vi "Script 3.vi"() -> ()   [LabVIEW 2020]
uses:
  <vilib>/Utility/miscctls.llb/LVRectTypeDef.ctl
  <vilib>/Utility/miscctls.llb/LVPositionTypeDef.ctl
  _csmHelper/CSM-Helper.lvclass/CSM-Helper.ctl
  _csmHelper/Properties/Read Case Structure Ref.vi
  _csmHelper/API/Create From VI Reference.vi
  _csmHelper/API/Start Undo.vi
  _csmHelper/Properties/Read Block Diagram Ref.vi
  _csmHelper/API/Destroy.vi
  _csmHelper/API/Connect StateQ Wire If not Connected.vi
  _csmHelper/API/Connect Internal Data Wire If not Connected.vi
  _csmHelper/API/Set Error Tunnel Use Default If not Connected.vi
  _csmHelper/API/Get CaseFrame Reference By CaseName.vi
  _csmHelper/API/Stop Undo.vi
  _csmHelper/CSM-Helper.lvclass
panel:
  in  "Top":i16
  in  "Left":i16
  out "Bounds:Area Height 2":u32
  out "Bounds:Area Width 2":u32
  out "Bounds:Area Width":u32
  out "Bounds:Area Height":u32
  in  "element":string="UI: Cursor Set"
  out "index of element":i32[](array[numeric])
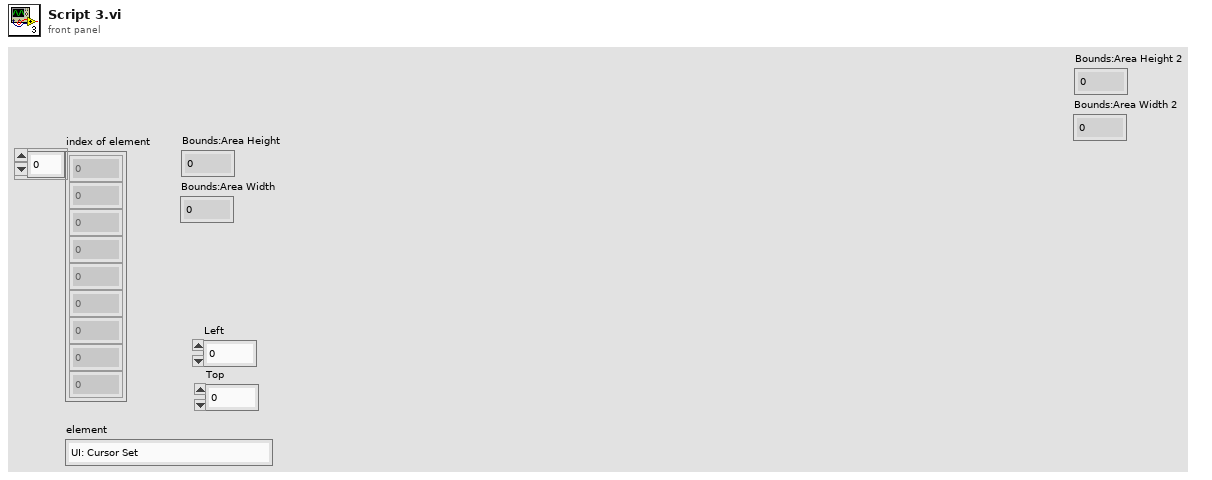
[diagram p1: front panel]
types:
  T1 = typedef "LVPositionTypeDef.ctl" = cluster{"Left":i32, "Top":i32}
  T2 = typedef "LVRectTypeDef.ctl" = cluster{"Left":i16, "Top":i16, "Right":i16, "Bottom":i16}
  T3 = cluster{"InternalData":refnum<vi>, "CSM Name":refnum<vi>, "Last Resp":refnum<vi>, "Remaining State":refnum<vi>, "Arguments":refnum<vi>, "Response Source":refnum<vi>, "Source CSM":refnum<vi>, "Selector":refnum<vi>, "Error":refnum<vi>}
  T4 = cluster{"InternalData":refnum<vi>, "Resp":refnum<vi>, "Remaining State":refnum<vi>, "Error":refnum<vi>}
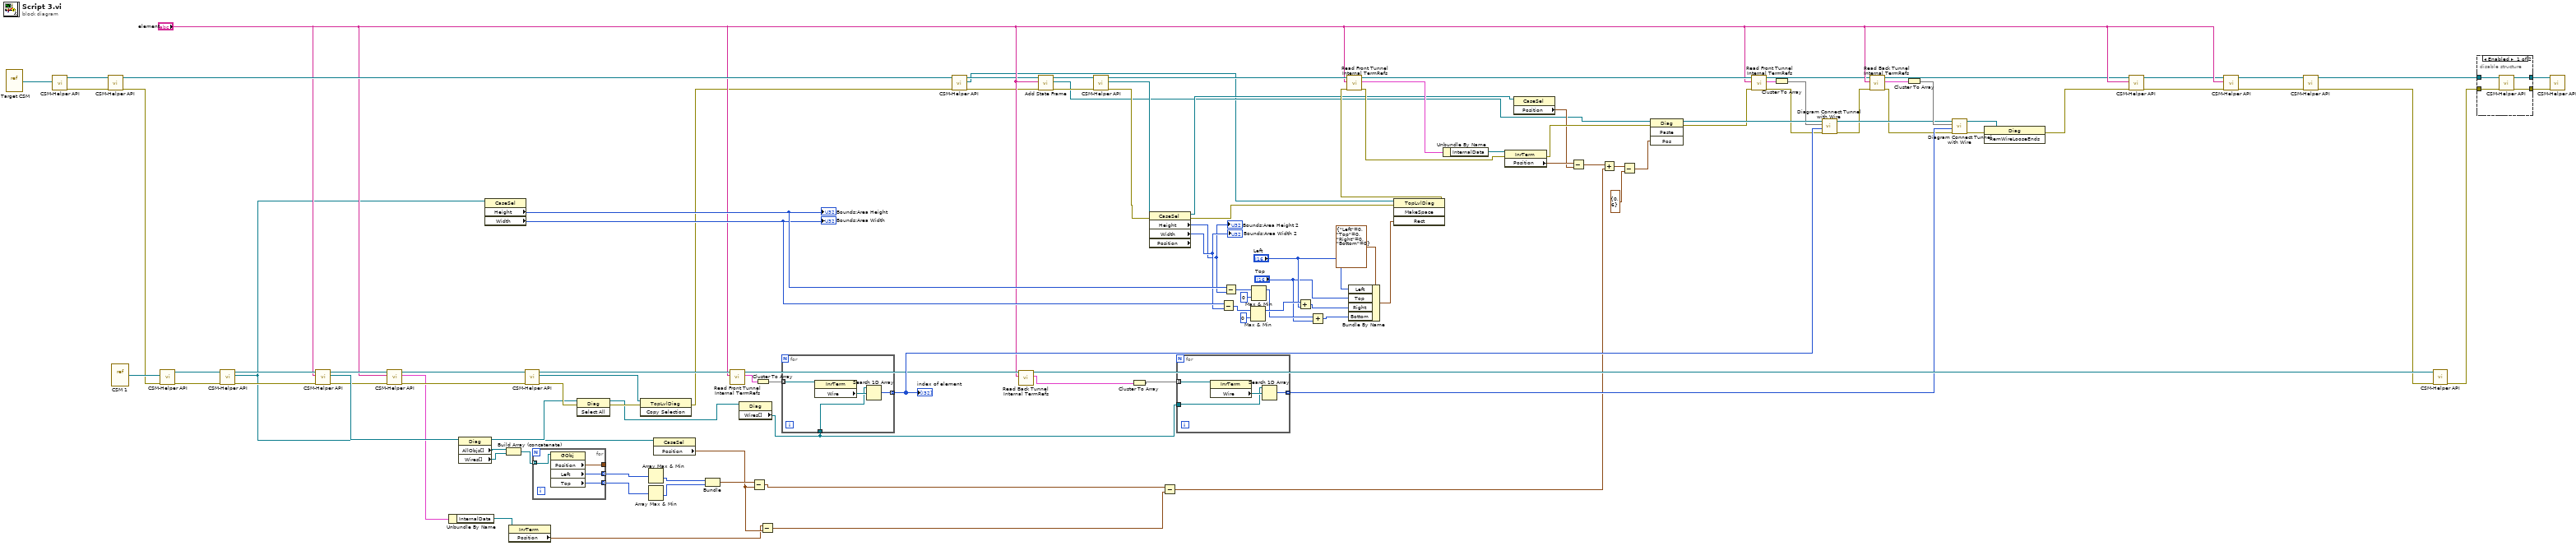
[diagram p0: block diagram]
diagram:
  n1 = vi-ref "Target CSM.vi"() -> (w110:refnum<vi>)
  n2 = call-poly "CSM-Helper API.vi"("VI"=w110) -> ("error out"=w109:errorcluster, "CSM-Helper.lvclass"=w108:refnum<class "CSM-Helper.lvclass">)  [unwired: 9 in]
  n3 = call-poly "CSM-Helper API.vi"("error in (no error)"=w109, "CSM-Helper in"=w108) -> ("error out"=w99:errorcluster, "CSM-Helper out"=w107:refnum<class "CSM-Helper.lvclass">)  [unwired: 8 in]
  n4 = vi-ref "CSM 1.vi"() -> (w111:refnum<vi>)
  n5 = call-poly "CSM-Helper API.vi"("error in (no error)"=w99, "VI"=w111) -> ("error out"=w102:errorcluster, "CSM-Helper.lvclass"=w103:refnum<class "CSM-Helper.lvclass">)  [unwired: 8 in]
  n6 = call-poly "CSM-Helper API.vi"("error in (no error)"=w102, "CSM-Helper in"=w103) -> ("error out"=w62:errorcluster, "Case Structure"=w31:refnum<vi>, "CSM-Helper out"=w63:refnum<class "CSM-Helper.lvclass">)  [unwired: 7 in]
  n7 = call-poly "CSM-Helper API.vi"("error in (no error)"=w62, "CASE"="element", "CSM-Helper in"=w63) -> ("error out"=w41:errorcluster, "Frame Refs"=w78:refnum<vi>, "CSM-Helper out"=w44:refnum<class "CSM-Helper.lvclass">)  [unwired: 6 in]
  n8 = call-poly "CSM-Helper API.vi"("error in (no error)"=w41, "case"="element", "CSM-Helper in"=w44) -> ("error out"=w40:errorcluster, "Front Tunnels"=w39:T3, "CSM-Helper out"=w43:refnum<class "CSM-Helper.lvclass">)  [unwired: 6 in]
  n9 = Unbundle By Name(w39) -> ("InternalData"=w38:refnum<vi>)
  n10 = property class="Diag"(reference=w78) -> (reference out=w46:refnum<vi>, "AllObjs[]"=w52:refnum<vi>[], "Wires[]"=w51:refnum<vi>[])  [unwired: 1 in, 1 out]
  n11 = property class="CaseSel"(reference=w31) -> ("Height"=w77:u32, "Width"=w76:u32)  [unwired: 1 in, 2 out]
  "Bounds:Area Height" <- w77
  "Bounds:Area Width" <- w76
  n12 = Build Array (concatenate)(w52, w51) -> (w50:refnum<vi>[])
  n13 = property class="InrTerm"(reference=w38) -> ("Position"=w29:T1)  [unwired: 1 in, 2 out]
  n14 = call-poly "CSM-Helper API.vi"("error in (no error)"=w40, "CSM-Helper in"=w43) -> ("error out"=w98:errorcluster, "Diagram"=w94:refnum<vi>, "CSM-Helper out"=w86:refnum<class "CSM-Helper.lvclass">)  [unwired: 7 in]
  n15 = for {
    tunnel: w50 -> [w115] mode=indexing
    tunnel: [w114] -> w53 mode=indexing
    tunnel: [w113] -> w54 mode=indexing
    tunnel: [w112] -> _
    n16 = property class="GObj"(reference=w115) -> ("Position"=w112:T1, "Left"=w114:i32, "Top"=w113:i32)  [unwired: 1 in, 2 out]
  }
  n17 = invoke class="Diag" method="Select All"(reference=w46, error in=w98) -> (reference out=w57:refnum<vi>, error out=w97:errorcluster)  [unwired: 1 in, 1 out]
  n18 = invoke class="TopLvlDiag" method="Copy Selection"(reference=w94, error in=w97) -> (error out=w8:errorcluster)  [unwired: 1 in, 2 out]
  n19 = Array Max & Min(array=w53) -> (min value=w49:i32)  [unwired: 3 out]
  n20 = Array Max & Min(array=w54) -> (min value=w48:i32)  [unwired: 3 out]
  n21 = property class="CaseSel"(reference=w31) -> ("Position"=w30:T1)  [unwired: 1 in, 2 out]
  n22 = Bundle(w49, w48) -> (w45:cluster{i32, i32})  [unwired: 1 in]
  n23 = call "Read Front Tunnel Internal TermRefs.vi"("case"="element", "CSM-Helper in"=w86) -> ("Front Tunnels"=w92:T3, "CSM-Helper out"=w85:refnum<class "CSM-Helper.lvclass">)  [unwired: 7 in, 1 out]
  n24 = property class="Diag"(reference=w57) -> ("Wires[]"=w56:refnum<vi>[])  [unwired: 1 in, 2 out]
  n25 = Subtract(x=w45, y=w30) -> (x-y=w37:T1)
  n26 = Cluster To Array(cluster=w92) -> (array=w91:refnum<vi>[])
  n27 = Subtract(x=w29, y=w30) -> (x-y=w27:T1)
  n28 = for {
    tunnel: w56 -> [w118]
    tunnel: [w117] -> w93 mode=indexing
    tunnel: w91 -> [w116] mode=indexing
    n29 = property class="InrTerm"(reference=w116) -> ("Wire"=w119:refnum<vi>)  [unwired: 1 in, 2 out]
    n30 = Search 1D Array(1D array=w118, element=w119) -> (index of element=w117:i32)  [unwired: 1 in]
  }
  "index of element" <- w93
  n31 = call-poly "CSM-Helper API.vi"("error in (no error)"=w8, "CSM-Helper in"=w107) -> ("error out"=w7:errorcluster, "Diagram"=w1:refnum<vi>, "CSM-Helper out"=w9:refnum<class "CSM-Helper.lvclass">)  [unwired: 7 in]
  n32 = call "Read Back Tunnel Internal TermRefs.vi"("element"="element", "CSM-Helper in"=w85) -> ("Front Tunnels"=w82:T4, "CSM-Helper out"=w84:refnum<class "CSM-Helper.lvclass">)  [unwired: 7 in, 1 out]
  n33 = call "Add State Frame.vi"("error in (no error)"=w7, "element"="element", "CSM-Helper in"=w9) -> ("error out"=w60:errorcluster, "Add Frame"=w6:refnum<vi>, "CSM-Helper out"=w100:refnum<class "CSM-Helper.lvclass">)  [unwired: 6 in]
  n34 = call-poly "CSM-Helper API.vi"("error in (no error)"=w60, "CSM-Helper in"=w100) -> ("error out"=w59:errorcluster, "Case Structure"=w58:refnum<vi>, "CSM-Helper out"=w61:refnum<class "CSM-Helper.lvclass">)  [unwired: 7 in]
  n35 = Cluster To Array(cluster=w82) -> (array=w83:refnum<vi>[])
  n36 = property class="CaseSel" props=["Height", "Width", "Position"](reference=w58, error in=w59) -> (reference out=w35:refnum<vi>, error out=w64:errorcluster, "Height"=w68:u32, "Width"=w69:u32)  [unwired: 1 out]
  "Bounds:Area Height 2" <- w68
  "Bounds:Area Width 2" <- w69
  n37 = Subtract(x=w37, y=w27) -> (x-y=w28:T1)
  n38 = for {
    tunnel: w56 -> [w122]
    tunnel: [w121] -> w81 mode=indexing
    tunnel: w83 -> [w120] mode=indexing
    n39 = property class="InrTerm"(reference=w120) -> ("Wire"=w123:refnum<vi>)  [unwired: 1 in, 2 out]
    n40 = Search 1D Array(1D array=w122, element=w123) -> (index of element=w121:i32)  [unwired: 1 in]
  }
  n41 = Subtract(x=w76, y=w69) -> (x-y=w71:u32)
  n42 = Subtract(x=w77, y=w68) -> (x-y=w74:u32)
  n43 = Max & Min(x=w71, y=u32 0) -> (max(x,y)=w67:u32)  [unwired: 1 out]
  n44 = Max & Min(x=w74, y=u32 0) -> (max(x,y)=w66:u32)  [unwired: 1 out]
  n45 = Add(x=w67, y="Left") -> (x+y=w4:u32)
  n46 = Add(x=w66, y="Top") -> (x+y=w5:u32)
  n47 = Bundle By Name(cluster=T2 {"Left"=0, "Top"=0, "Right"=0, "Bottom"=0} ("Rect"), "Left"="Left", "Top"="Top", "Right"=w4, "Bottom"=w5) -> (w70:T2)
  n48 = invoke class="TopLvlDiag" method="MakeSpace"(reference=w1, error in=w64, "Rect"=w70) -> (error out=w65:errorcluster)  [unwired: 1 in, 3 out]
  n49 = call "Read Front Tunnel Internal TermRefs.vi"("error in (no error)"=w65, "case"="element", "CSM-Helper in"=w61) -> ("error out"=w95:errorcluster, "Front Tunnels"=w90:T3, "CSM-Helper out"=w88:refnum<class "CSM-Helper.lvclass">)  [unwired: 6 in]
  n50 = Unbundle By Name(w90) -> ("InternalData"=w101:refnum<vi>)
  n51 = property class="InrTerm"(reference=w101, error in=w95) -> (error out=w96:errorcluster, "Position"=w36:T1)  [unwired: 1 out]
  n52 = property class="CaseSel"(reference=w35) -> ("Position"=w34:T1)  [unwired: 1 in, 2 out]
  n53 = Subtract(x=w36, y=w34) -> (x-y=w55:T1)
  n54 = Add(x=w55, y=w28) -> (x+y=w47:T1)
  n55 = Subtract(x=w47, y=T1 {"Left"=0, "Top"=6}) -> (x-y=w33:T1)
  n56 = invoke class="Diag" method="Paste"(reference=w6, error in=w96, "Pos"=w33) -> (reference out=w89:refnum<vi>, error out=w87:errorcluster)  [unwired: 1 in, 2 out]
  n57 = call "Read Front Tunnel Internal TermRefs.vi"("error in (no error)"=w87, "case"="element", "CSM-Helper in"=w88) -> ("error out"=w25:errorcluster, "Front Tunnels"=w24:T3, "CSM-Helper out"=w22:refnum<class "CSM-Helper.lvclass">)  [unwired: 6 in]
  n58 = Cluster To Array(cluster=w24) -> (array=w26:refnum<vi>[])
  n59 = call "Diagram Connect Tunnel with Wire.vi"("error in (no error)"=w25, "Wire Indexs"=w93, "Front Tunnels"=w26, "Diagram in"=w89) -> ("error out"=w15:errorcluster, "Diagram out"=w17:refnum<vi>)  [unwired: 5 in, 1 out]
  n60 = call "Read Back Tunnel Internal TermRefs.vi"("error in (no error)"=w15, "element"="element", "CSM-Helper in"=w22) -> ("error out"=w14:errorcluster, "Front Tunnels"=w23:T4, "CSM-Helper out"=w21:refnum<class "CSM-Helper.lvclass">)  [unwired: 6 in]
  n61 = Cluster To Array(cluster=w23) -> (array=w18:refnum<vi>[])
  n62 = call "Diagram Connect Tunnel with Wire.vi"("error in (no error)"=w14, "Wire Indexs"=w81, "Front Tunnels"=w18, "Diagram in"=w17) -> ("error out"=w16:errorcluster, "Diagram out"=w10:refnum<vi>)  [unwired: 5 in, 1 out]
  n63 = invoke class="Diag" method="RemWireLooseEnds"(reference=w10, error in=w16) -> (error out=w11:errorcluster)  [unwired: 1 in, 2 out]
  n64 = call-poly "CSM-Helper API.vi"("error in (no error)"=w11, "case"="element", "CSM-Helper in"=w21) -> ("error out"=w20:errorcluster, "CSM-Helper out"=w19:refnum<class "CSM-Helper.lvclass">)  [unwired: 7 in]
  n65 = call-poly "CSM-Helper API.vi"("error in (no error)"=w20, "case"="element", "CSM-Helper in"=w19) -> ("error out"=w12:errorcluster, "CSM-Helper out"=w13:refnum<class "CSM-Helper.lvclass">)  [unwired: 7 in]
  n66 = call-poly "CSM-Helper API.vi"("error in (no error)"=w12, "CSM-Helper in"=w13) -> ("error out"=w79:errorcluster, "CSM-Helper out"=w80:refnum<class "CSM-Helper.lvclass">)  [unwired: 8 in]
  n67 = call-poly "CSM-Helper API.vi"("error in (no error)"=w79, "CSM-Helper in"=w84) -> ("error out"=w105:errorcluster)  [unwired: 8 in, 1 out]
  n68 = disable-structure shown="Enabled" {
    disable-tunnel: [w127 w129] -> w106
    disable-tunnel: w105 -> [w126 w128]
    disable-tunnel: [w125 w128] -> w104
    disable-tunnel: w80 -> [w124 w129]
    frame Enabled {
      n69 = call-poly "CSM-Helper API.vi"("error in (no error)"=w126, "CSM-Helper in"=w124) -> ("error out"=w125:errorcluster, "CSM-Helper out"=w127:refnum<class "CSM-Helper.lvclass">)  [unwired: 8 in]
    }
    frame Disabled {
    }
  }
  n70 = call-poly "CSM-Helper API.vi"("error in (no error)"=w104, "CSM-Helper in"=w106) -> ()  [unwired: 8 in, 2 out]
